vi "rdb_json_next_char.vi"(10 "offset (0)":i32, 11 "json":string) -> (2 "offset before char":i32, 3 "non-whitespace char":string)   [LabVIEW 2017]
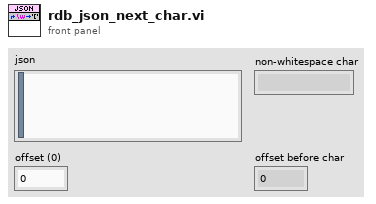
[diagram p1: front panel]
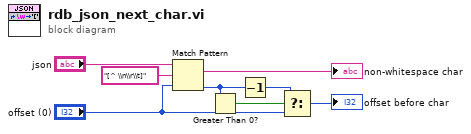
[diagram p0: block diagram]
diagram:
  n1 = Match Pattern(string="json", regular expression="[^ \\n\\r\\t]", offset (0)="offset (0)") -> (match substring=→"non-whitespace char":string, offset past match=w4:i32)  [unwired: 2 out]
  n2 = Greater Than 0?(x=w4) -> (x > 0?=w6:bool)
  n3 = Decrement(x=w4) -> (x-1=w1:i32)
  n4 = Select(t=w1, s=w6, f="offset (0)") -> (s? t:f=→"offset before char":i32)
